vi "Swerve Drive Straight.vi"(0 "Xin":dbl, 3 "Yin":dbl) -> (7 "Xout":dbl, 10 "Yout":dbl)   [LabVIEW 2016]
uses:
  <vilib>/Rock Robotics/WPI/ThirdParty/CanMotor/TalonSRX/WPI_CANTalonSRX_APIControlMode.ctl
  Robot Global Data.vi
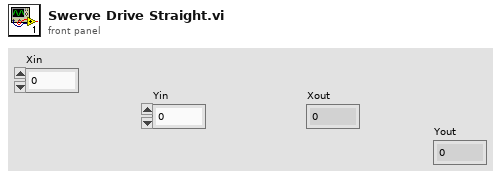
[diagram p1: front panel]
types:
  T1 = enum16{"Start setup globals", "Setup Position control", "run the pid loop", "Change the mode back to PWM", "Finish return values to default"}
  T2 = enum16{"Can ID", "P", "I", "D", "F", "IZone", "RampSpeed", "Fwd speed Limit", "Rev Speed Limit", "InvertDrive"}
  T3 = enum16{"FL Drive Wheel", "FR Drive Wheel", "RL Drive Wheel", "RR Drive Wheel", "FL Steer Wheel", "FR Steer Wheel", "RL Steer Wheel", "RR Steer Wheel"}
  T4 = typedef "WPI_CANTalonSRX_APIControlMode.ctl" = enum8{"Percent VBus", "Speed", "Position", "Slave", "Unchanged / Invalid", "Voltage Compensation", "Current", "Motion Profile", "Motion Magic"}
  T5 = typedef "WPI_MotorControlDeviceRef.ctl" = cluster{"DeviceStatus":errorcluster, "Type":T6, "PWM":cluster{"PWM Channel":T7, "DeadBand":T8}, "CAN":cluster{"Device Number":u8, "SetOutput VI Ref":variant, "GetOutput VI Ref":variant, "Enable VI Ref":variant, "Disable VI Ref":variant, "Data":variant}, "Invert":bool}
  T6 = typedef "WPI_MotorControlType.ctl" = enum16{"PWM", "CAN"}
  T7 = typedef "FPGA_DIOPWMChannel.ctl" = enum8{"PWM 0", "PWM 1", "PWM 2", "PWM 3", "PWM 4", "PWM 5", "PWM 6", "PWM 7", "PWM 8", "PWM 9", "PWM MXP 0", "PWM MXP 1", "PWM MXP 2", "PWM MXP 3", "PWM MXP 4", "PWM MXP 5", "PWM MXP 6", "PWM MXP 7", "PWM MXP 8", "PWM MXP 9", "Invalid"}
  T8 = typedef "WPI_PWMDeadband.ctl" = cluster{"Name":string, "maxPositivePwm":i32, "minPositivePwm":i32, "centerPwm":i32, "maxNegativePwm":i32, "minNegativePwm":i32, "angularRange":u16}
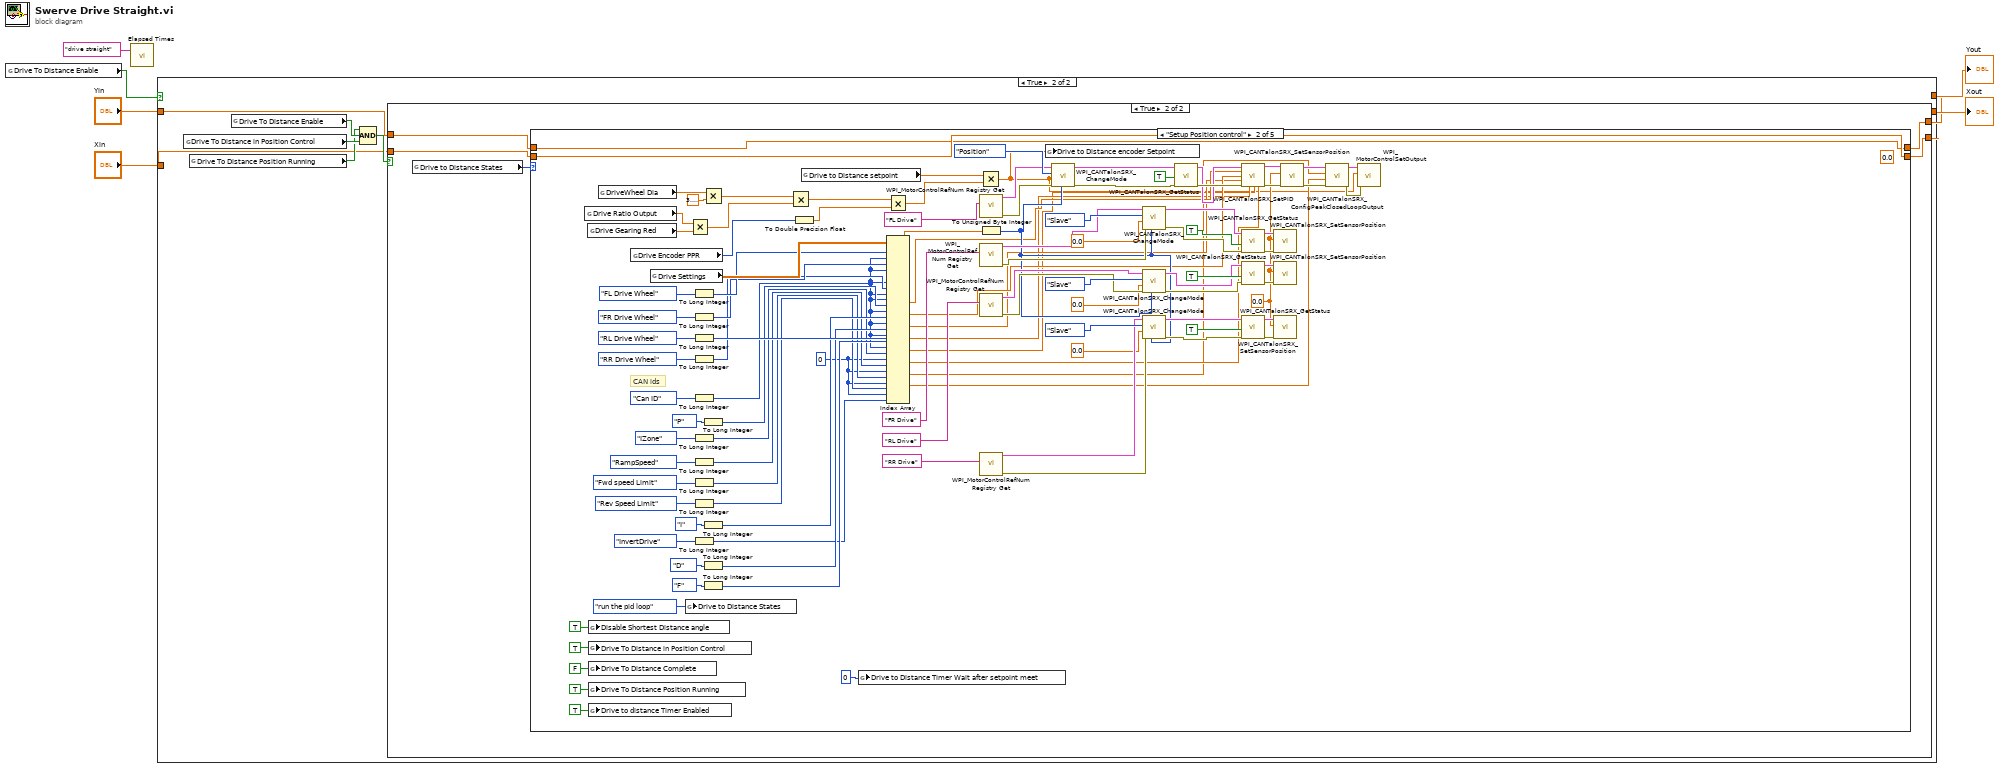
[diagram p0: block diagram]
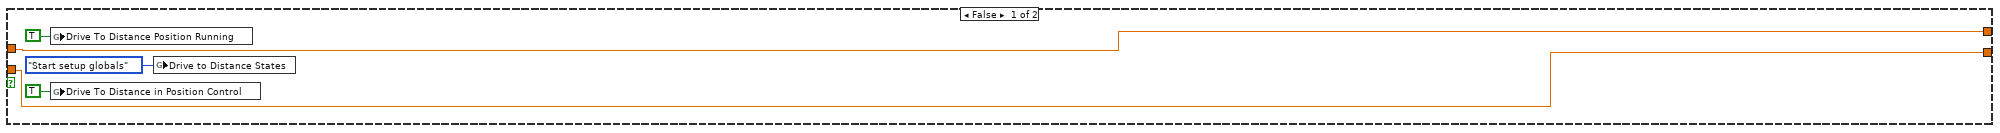
[diagram p3: hidden frame]
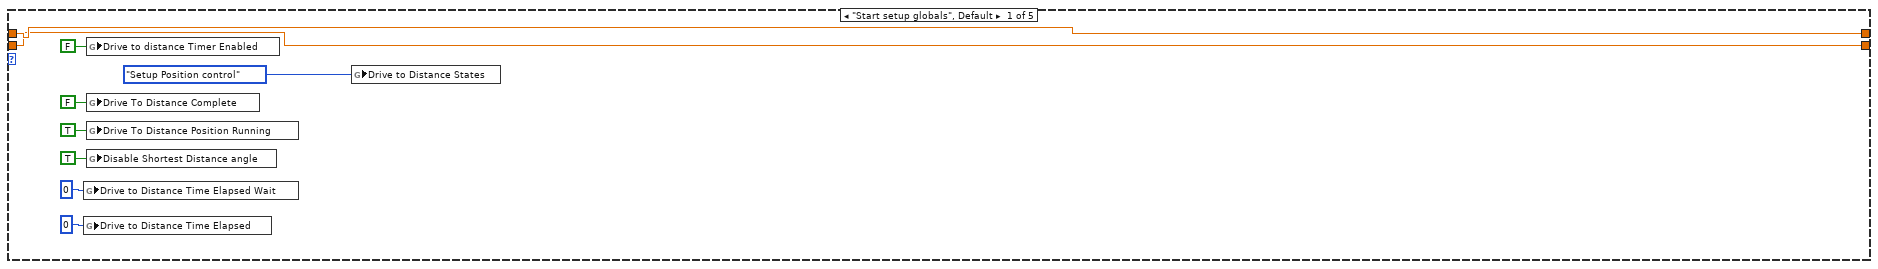
[diagram p4: hidden frame]
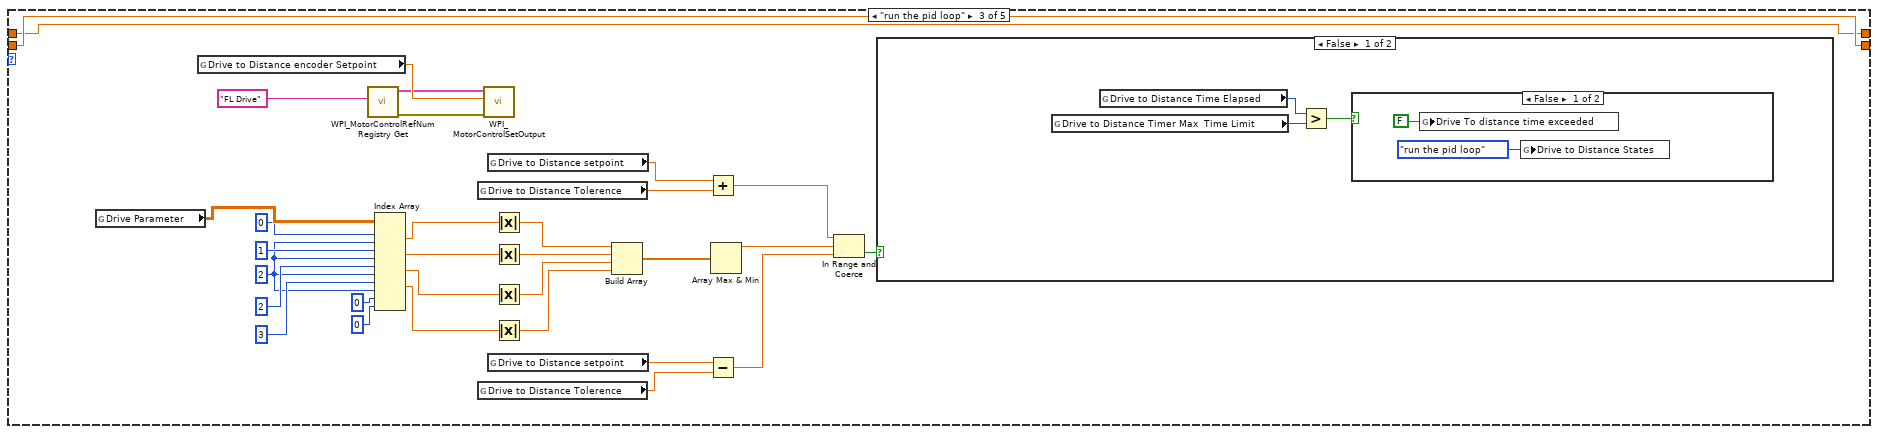
[diagram p5: hidden frame]
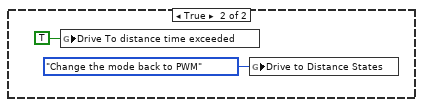
[diagram p6: hidden frame]
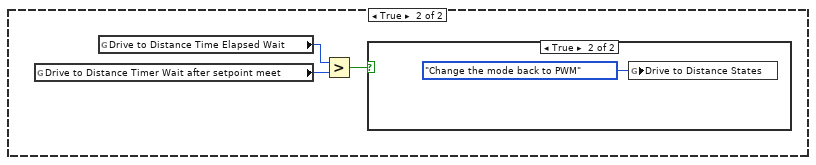
[diagram p7: hidden frame]
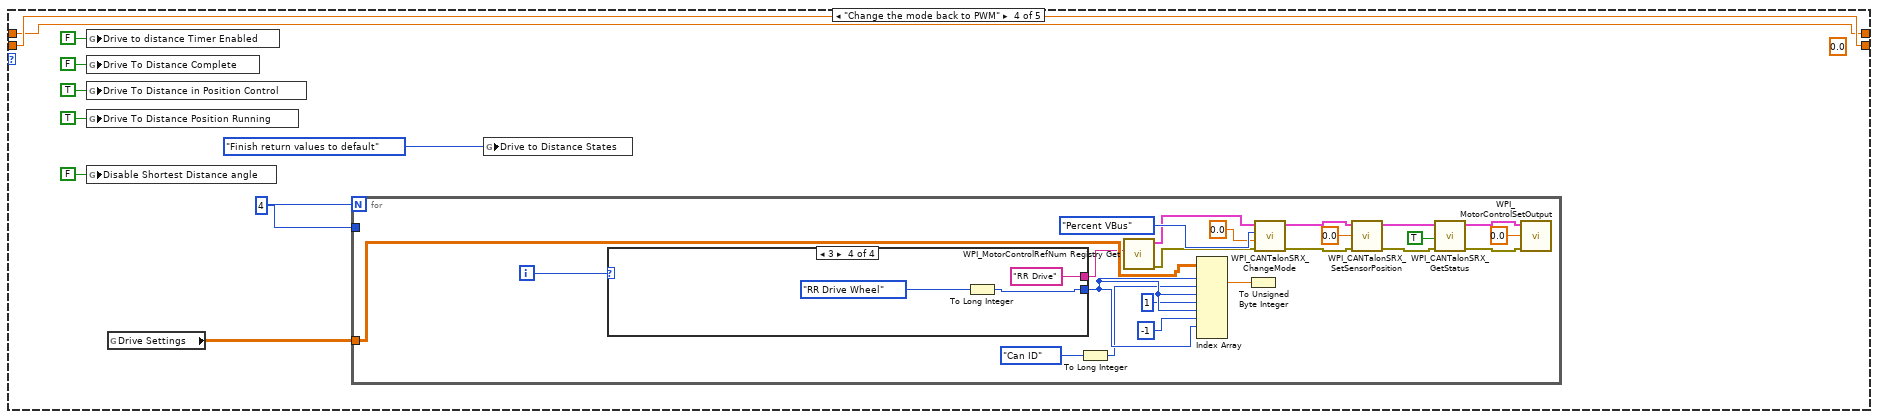
[diagram p9: hidden frame]
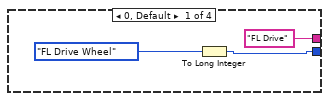
[diagram p10: hidden frame]
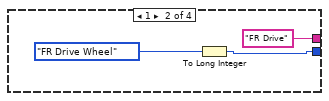
[diagram p11: hidden frame]
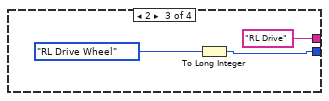
[diagram p12: hidden frame]
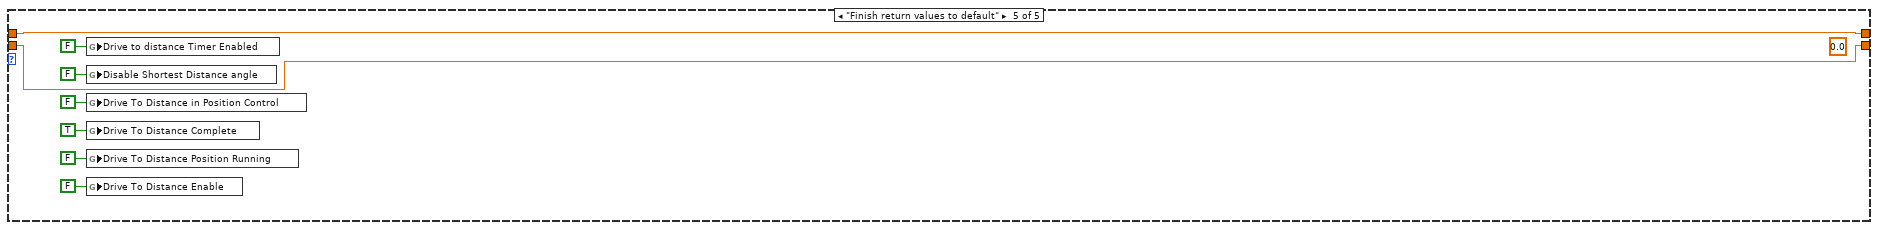
[diagram p13: hidden frame]
diagram:
  n1 = global read "Robot Global Data.vi" "Drive To Distance Enable"() -> (w2:bool)
  n2 = call "Elapsed Times.vi"("Call Name"="drive straight") -> ()  [unwired: 2 in, 1 out]
  n3 = case shown="True" w2 {
    tunnel: [w8 w10] -> w4
    tunnel: "Xin" -> [w8 w12]
    tunnel: [w7 w9] -> w3
    tunnel: "Yin" -> [w7 w11]
    frame False {
    }
    frame True {
      n4 = global read "Robot Global Data.vi" "Drive To Distance in Position Control"() -> (w16:bool)
      n5 = global read "Robot Global Data.vi" "Drive To Distance Position Running"() -> (w14:bool)
      n6 = global read "Robot Global Data.vi" "Drive To Distance Enable"() -> (w15:bool)
      n7 = Compound Arithmetic op=AND(w14, w15, w16) -> (w13:bool)
      n8 = case shown="True" w13 {
        tunnel: w12 -> [w18 w25]
        tunnel: w11 -> [w17 w24]
        tunnel: [w18 w22] -> w10
        tunnel: [w17 w23] -> w9
        frame False {
          n9 = global write "Robot Global Data.vi" "Drive To Distance Position Running"(TRUE ("Drive To Distance Position Running")) -> ()
          n10 = global write "Robot Global Data.vi" "Drive To Distance in Position Control"(TRUE ("Drive To Distance in Position Control")) -> ()
          n11 = global write "Robot Global Data.vi" "Drive to Distance States"(T1."Start setup globals" ("Drive to Distance States")) -> ()
        }
        frame True {
          n12 = global read "Robot Global Data.vi" "Drive to Distance States"() -> (w26:T1)
          n13 = case shown="\"Setup Position control\"" w26 {
            tunnel: w25 -> [w27 w38 w144 w187 w231]
            tunnel: w24 -> [w28 w37 w143 w186 w230]
            tunnel: [w28 w37 w143 w186 w230] -> w23
            tunnel: [w27 w38 w144 w187 w231] -> w22
            frame "Start setup globals", Default {
              n14 = global write "Robot Global Data.vi" "Drive to Distance Time Elapsed Wait"(u32 0 ("Drive to Distance Time Elapsed Wait")) -> ()
              n15 = global write "Robot Global Data.vi" "Drive to Distance Time Elapsed"(u32 0 ("Drive to Distance Time Elapsed")) -> ()
              n16 = global write "Robot Global Data.vi" "Drive to distance Timer Enabled"(FALSE ("Drive To Distance in Position Control")) -> ()
              n17 = global write "Robot Global Data.vi" "Drive To Distance Complete"(FALSE ("Drive To Distance Complete")) -> ()
              n18 = global write "Robot Global Data.vi" "Drive To Distance Position Running"(TRUE ("Drive To Distance Position Running")) -> ()
              n19 = global write "Robot Global Data.vi" "Disable Shortest Distance angle"(TRUE ("Disable Shortest Distance angle")) -> ()
              n20 = global write "Robot Global Data.vi" "Drive to Distance States"(T1."Setup Position control" ("Drive to Distance States")) -> ()
            }
            frame "Setup Position control" {
              (unwired) 0.0 ("Numeric")
              w59 = 0.0 ("New Sensor Position")
              w80 = 0 ("index (row)")
              # "CAN ids"
              n21 = global read "Robot Global Data.vi" "Drive Ratio Output"() -> (w56:dbl)
              n22 = global read "Robot Global Data.vi" "Drive Gearing Red"() -> (w55:dbl)
              n23 = global write "Robot Global Data.vi" "Disable Shortest Distance angle"(TRUE ("Disable Shortest Distance angle")) -> ()
              n24 = global write "Robot Global Data.vi" "Drive To Distance in Position Control"(TRUE ("Drive To Distance in Position Control")) -> ()
              n25 = global write "Robot Global Data.vi" "Drive To Distance Complete"(FALSE ("Drive To Distance Complete")) -> ()
              n26 = global write "Robot Global Data.vi" "Drive To Distance Position Running"(TRUE ("Drive To Distance Position Cont")) -> ()
              n27 = global write "Robot Global Data.vi" "Drive to distance Timer Enabled"(TRUE ("Drive To Distance in Position Control")) -> ()
              n28 = global read "Robot Global Data.vi" "DriveWheel Dia"() -> (w54:dbl)
              n29 = global read "Robot Global Data.vi" "Drive Encoder PPR"() -> (w50:u32)
              n30 = global read "Robot Global Data.vi" "Drive Settings"() -> (w111:dbl[][])
              n31 = global write "Robot Global Data.vi" "Drive to Distance States"(T1."run the pid loop" ("Drive to Distance States")) -> ()
              n32 = Multiply(x=w56, y=w55) -> (x*y=w51:dbl)
              n33 = To Long Integer(number=T3."FL Drive Wheel" ("Swerve Drive Param")) -> (32bit integer=w99:i32)
              n34 = To Long Integer(number=T3."FR Drive Wheel" ("Swerve Drive Param")) -> (32bit integer=w97:i32)
              n35 = To Long Integer(number=T3."RL Drive Wheel" ("Swerve Drive Param")) -> (32bit integer=w98:i32)
              n36 = To Long Integer(number=T3."RR Drive Wheel" ("Swerve Drive Param")) -> (32bit integer=w96:i32)
              n37 = To Long Integer(number=T2."Can ID" ("Enum")) -> (32bit integer=w81:i32)
              n38 = To Long Integer(number=T2."IZone" ("Enum")) -> (32bit integer=w85:i32)
              n39 = To Long Integer(number=T2."RampSpeed" ("Enum")) -> (32bit integer=w86:i32)
              n40 = To Long Integer(number=T2."Fwd speed Limit" ("Enum")) -> (32bit integer=w84:i32)
              n41 = To Long Integer(number=T2."Rev Speed Limit" ("Enum")) -> (32bit integer=w82:i32)
              n42 = To Long Integer(number=T2."InvertDrive" ("Enum")) -> (32bit integer=w83:i32)
              n43 = To Long Integer(number=T2."D" ("Enum")) -> (32bit integer=w93:i32)
              n44 = To Long Integer(number=T2."F" ("Enum")) -> (32bit integer=w92:i32)
              n45 = Multiply(x=w54, y=3.141592653589793) -> (x*y=w52:dbl)
              n46 = To Long Integer(number=T2."P" ("Enum")) -> (32bit integer=w95:i32)
              n47 = To Long Integer(number=T2."I" ("Enum")) -> (32bit integer=w94:i32)
              n48 = Multiply(x=w52, y=w51) -> (x*y=w48:dbl)
              n49 = To Double Precision Float(number=w50) -> (double precision float=w49:dbl)
              n50 = global read "Robot Global Data.vi" "Drive to Distance setpoint"() -> (w46:dbl)
              n51 = global write "Robot Global Data.vi" "Drive to Distance Timer Wait after setpoint meet"(u32 0 ("Drive to Distance Timer Wait after setpoint meet")) -> ()
              n52 = Multiply(x=w48, y=w49) -> (x*y=w47:dbl)
              n53 = Index Array(array=w111, index (row) #1=w99, index (col) #1=w81, index (row) #2=w97, index (col) #2=w81, index (row) #3=w98, index (col) #3=w81, index (row) #4=w96, index (col) #4=w81, index (row) #5=w81, index (col) #5=w95, index (row) #6=w81, index (col) #6=w94, index (row) #7=w81, index (col) #7=w93, index (row) #8=w81, index (col) #8=w92, index (row) #9=w81, index (col) #9=w85, index (row) #10=w80, index (col) #10=w86, index (row) #11=w80, index (col) #11=w84, index (row) #12=w80, index (col) #12=w82, index (row) #13=w80, index (col) #13=w83) -> (element #1=w115:dbl, element #5=w79:dbl, element #6=w78:dbl, element #7=w77:dbl, element #8=w76:dbl, element #9=w75:dbl, element #10=w72:dbl, element #11=w69:dbl, element #12=w68:dbl)  [unwired: 4 out]
              n54 = Multiply(x=w46, y=w47) -> (x*y=w39:dbl)
              n55 = To Unsigned Byte Integer(number=w115) -> (unsigned 8bit integer=w114:u8)
              n56 = call <vilib>:"WPI_MotorControlRefNum Registry Get.vi"("refnum name"="FL Drive") -> ("error out"=w129:errorcluster, "MotorControlDevRef"=w133:T5)  [unwired: 9 in]
              n57 = call <vilib>:"WPI_MotorControlRefNum Registry Get.vi"("refnum name"="FR Drive") -> ("error out"=w128:errorcluster, "MotorControlDevRef"=w132:T5)  [unwired: 9 in]
              n58 = call <vilib>:"WPI_MotorControlRefNum Registry Get.vi"("refnum name"="RL Drive") -> ("error out"=w127:errorcluster, "MotorControlDevRef"=w131:T5)  [unwired: 9 in]
              n59 = call <vilib>:"WPI_MotorControlRefNum Registry Get.vi"("refnum name"="RR Drive") -> ("error out"=w126:errorcluster, "MotorControlDevRef"=w130:T5)  [unwired: 9 in]
              n60 = global write "Robot Global Data.vi" "Drive to Distance encoder Setpoint"(w39) -> ()
              n61 = call <vilib>:"WPI_CANTalonSRX_ChangeMode.vi"("Master Device Number"=w114, "error in (no error)"=w129, "Output"=w39, "Control Mode"=WPI_CANTalonSRX_APIControlMode."Position", "CAN Talon SRX Ref"=w133) -> ("error out"=w125:errorcluster, "CAN Talon SRX Ref"=w124:T5)  [unwired: 5 in]
              n62 = call <vilib>:"WPI_CANTalonSRX_ChangeMode.vi"("Master Device Number"=w114, "error in (no error)"=w128, "Output"=0.0, "Control Mode"=WPI_CANTalonSRX_APIControlMode."Slave", "CAN Talon SRX Ref"=w132) -> ("error out"=w109:errorcluster, "CAN Talon SRX Ref"=w110:T5)  [unwired: 5 in]
              n63 = call <vilib>:"WPI_CANTalonSRX_ChangeMode.vi"("Master Device Number"=w114, "error in (no error)"=w127, "Output"=0.0, "Control Mode"=WPI_CANTalonSRX_APIControlMode."Slave", "CAN Talon SRX Ref"=w131) -> ("error out"=w117:errorcluster, "CAN Talon SRX Ref"=w116:T5)  [unwired: 5 in]
              n64 = call <vilib>:"WPI_CANTalonSRX_ChangeMode.vi"("Master Device Number"=w114, "error in (no error)"=w126, "Output"=0.0, "Control Mode"=WPI_CANTalonSRX_APIControlMode."Slave", "CAN Talon SRX Ref"=w130) -> ("error out"=w118:errorcluster, "CAN Talon SRX Ref"=w119:T5)  [unwired: 5 in]
              n65 = call <vilib>:"WPI_CANTalonSRX_GetStatus.vi"("error in (no error)"=w125, "Clear Sticky Faults"=TRUE, "CAN Talon SRX Ref"=w124) -> ("error out"=w113:errorcluster, "CAN Talon SRX Ref"=w112:T5)  [unwired: 6 in, 1 out]
              n66 = call <vilib>:"WPI_CANTalonSRX_SetPID.vi"("CAN Talon SRX Ref"=w112, "P"=w79, "I"=w78, "D"=w77, "error in (no error)"=w113, "F"=w76, "I Zone"=w75, "Ramp Rate"=w72) -> ("CAN Talon SRX Ref"=w73:T5, "error out"=w74:errorcluster)  [unwired: 6 in]
              n67 = call <vilib>:"WPI_CANTalonSRX_GetStatus.vi"("error in (no error)"=w109, "Clear Sticky Faults"=TRUE, "CAN Talon SRX Ref"=w110) -> ("error out"=w60:errorcluster, "CAN Talon SRX Ref"=w61:T5)  [unwired: 6 in, 1 out]
              n68 = call <vilib>:"WPI_CANTalonSRX_GetStatus.vi"("error in (no error)"=w117, "Clear Sticky Faults"=TRUE, "CAN Talon SRX Ref"=w116) -> ("error out"=w62:errorcluster, "CAN Talon SRX Ref"=w63:T5)  [unwired: 6 in, 1 out]
              n69 = call <vilib>:"WPI_CANTalonSRX_GetStatus.vi"("error in (no error)"=w118, "Clear Sticky Faults"=TRUE, "CAN Talon SRX Ref"=w119) -> ("error out"=w64:errorcluster, "CAN Talon SRX Ref"=w65:T5)  [unwired: 6 in, 1 out]
              n70 = call <vilib>:"WPI_CANTalonSRX_SetSensorPosition.vi"("error in (no error)"=w60, "New Sensor Position"=w59, "CAN Talon SRX Ref"=w61) -> ()  [unwired: 7 in, 2 out]
              n71 = call <vilib>:"WPI_CANTalonSRX_SetSensorPosition.vi"("error in (no error)"=w62, "New Sensor Position"=w59, "CAN Talon SRX Ref"=w63) -> ()  [unwired: 7 in, 2 out]
              n72 = call <vilib>:"WPI_CANTalonSRX_SetSensorPosition.vi"("error in (no error)"=w64, "New Sensor Position"=w59, "CAN Talon SRX Ref"=w65) -> ()  [unwired: 7 in, 2 out]
              n73 = call <vilib>:"WPI_CANTalonSRX_SetSensorPosition.vi"("error in (no error)"=w74, "New Sensor Position"=w59, "CAN Talon SRX Ref"=w73) -> ("error out"=w71:errorcluster, "CAN Talon SRX Ref"=w70:T5)  [unwired: 7 in]
              n74 = call <vilib>:"WPI_CANTalonSRX_ConfigPeakClosedLoopOutput.vi"("error in (no error)"=w71, "Reverse Peak Output"=w68, "Forward Peak Output"=w69, "CAN Talon SRX Ref"=w70) -> ("error out"=w45:errorcluster, "CAN Talon SRX Ref"=w44:T5)  [unwired: 6 in]
              n75 = call <vilib>:"WPI_MotorControlSetOutput.vi"("error in (no error)"=w45, "Output"=w39, "MotorControlDevRef"=w44) -> ()  [unwired: 6 in, 3 out]
            }
            frame "run the pid loop" {
              w170 = 2 ("disabled index (col)")
              n76 = global read "Robot Global Data.vi" "Drive Parameter"() -> (w169:dbl[][])
              n77 = global read "Robot Global Data.vi" "Drive to Distance encoder Setpoint"() -> (w148:dbl)
              n78 = call <vilib>:"WPI_MotorControlRefNum Registry Get.vi"("refnum name"="FL Drive") -> ("error out"=w145:errorcluster, "MotorControlDevRef"=w146:T5)  [unwired: 9 in]
              n79 = Index Array(array=w169, index (row) #1=0 ("disabled index (row)"), index (col) #1=w170, index (row) #2=1 ("index (row)"), index (col) #2=w170, index (row) #3=2 ("index (row)"), index (col) #3=w170, index (row) #4=3 ("index (row)"), index (col) #4=w170, index (row) #5=0 ("index (row)"), index (col) #5=0 ("disabled index (col)")) -> (element #1=w167:dbl, element #2=w164:dbl, element #3=w165:dbl, element #4=w166:dbl)  [unwired: 1 out]
              n80 = global read "Robot Global Data.vi" "Drive to Distance Tolerence"() -> (w156:dbl)
              n81 = global read "Robot Global Data.vi" "Drive to Distance Tolerence"() -> (w154:dbl)
              n82 = call <vilib>:"WPI_MotorControlSetOutput.vi"("error in (no error)"=w145, "Output"=w148, "MotorControlDevRef"=w146) -> ()  [unwired: 6 in, 3 out]
              n83 = global read "Robot Global Data.vi" "Drive to Distance setpoint"() -> (w157:dbl)
              n84 = global read "Robot Global Data.vi" "Drive to Distance setpoint"() -> (w153:dbl)
              n85 = Absolute Value(x=w167) -> (abs(x)=w160:dbl)
              n86 = Absolute Value(x=w164) -> (abs(x)=w161:dbl)
              n87 = Absolute Value(x=w165) -> (abs(x)=w162:dbl)
              n88 = Absolute Value(x=w166) -> (abs(x)=w163:dbl)
              n89 = Build Array(w160, w161, w162, w163) -> (w159:dbl[])
              n90 = Add(x=w157, y=w156) -> (x+y=w155:dbl)
              n91 = Subtract(x=w153, y=w154) -> (x-y=w152:dbl)
              n92 = Array Max & Min(array=w159) -> (max value=w158:dbl)  [unwired: 3 out]
              n93 = In Range and Coerce(upper limit=w155, x=w158, lower limit=w152) -> (In Range?=w151:bool)  [unwired: 1 out]
              n94 = case shown="False" w151 {
                frame False {
                  n95 = global read "Robot Global Data.vi" "Drive to Distance Timer Max  Time Limit"() -> (w175:u32)
                  n96 = global read "Robot Global Data.vi" "Drive to Distance Time Elapsed"() -> (w176:u32)
                  n97 = Greater?(x=w176, y=w175) -> (0:w174:bool)
                  n98 = case shown="False" w174 {
                    frame False {
                      n99 = global write "Robot Global Data.vi" "Drive To distance time exceeded"(FALSE ("Drive To distance time exceeded")) -> ()
                      n100 = global write "Robot Global Data.vi" "Drive to Distance States"(T1."run the pid loop" ("Drive to Distance States")) -> ()
                    }
                    frame True {
                      n101 = global write "Robot Global Data.vi" "Drive To distance time exceeded"(TRUE ("Drive To distance time exceeded")) -> ()
                      n102 = global write "Robot Global Data.vi" "Drive to Distance States"(T1."Change the mode back to PWM" ("Drive to Distance States")) -> ()
                    }
                  }
                }
                frame True {
                  n103 = global read "Robot Global Data.vi" "Drive to Distance Timer Wait after setpoint meet"() -> (w182:u32)
                  n104 = global read "Robot Global Data.vi" "Drive to Distance Time Elapsed Wait"() -> (w183:u32)
                  n105 = Greater?(x=w183, y=w182) -> (0:w181:bool)
                  n106 = case shown="True" w181 {
                    frame False {
                    }
                    frame True {
                      n107 = global write "Robot Global Data.vi" "Drive to Distance States"(T1."Change the mode back to PWM" ("Drive to Distance States")) -> ()
                    }
                  }
                }
              }
            }
            frame "Change the mode back to PWM" {
              (unwired) 0.0 ("Numeric")
              w193 = 4
              n108 = global write "Robot Global Data.vi" "Drive to distance Timer Enabled"(FALSE ("Drive to distance Timer Enabled")) -> ()
              n109 = global write "Robot Global Data.vi" "Drive To Distance Complete"(FALSE ("Drive To Distance Complete")) -> ()
              n110 = global write "Robot Global Data.vi" "Drive To Distance in Position Control"(TRUE ("Drive To Distance in Position Control")) -> ()
              n111 = global write "Robot Global Data.vi" "Drive To Distance Position Running"(TRUE ("Drive To Distance Position Cont")) -> ()
              n112 = global write "Robot Global Data.vi" "Disable Shortest Distance angle"(FALSE ("Disable Shortest Distance angle")) -> ()
              n113 = global read "Robot Global Data.vi" "Drive Settings"() -> (w194:dbl[][])
              n114 = for {
                N: w193 -> [_]
                tunnel: w194 -> [w213]
                tunnel: w193 -> [_]
                i -> [w216]
                n115 = case shown="3" w216 {
                  tunnel: [w219 w221 w224 w227] -> w211
                  tunnel: ["FL Drive" ("refnum name") "FR Drive" ("refnum name") "RL Drive" ("refnum name") "RR Drive" ("refnum name")] -> w201
                  frame 0, Default {
                    n116 = To Long Integer(number=T3."FL Drive Wheel" ("Swerve Drive Param")) -> (32bit integer=w219:i32)
                  }
                  frame 1 {
                    n117 = To Long Integer(number=T3."FR Drive Wheel" ("Swerve Drive Param")) -> (32bit integer=w221:i32)
                  }
                  frame 2 {
                    n118 = To Long Integer(number=T3."RL Drive Wheel" ("Swerve Drive Param")) -> (32bit integer=w224:i32)
                  }
                  frame 3 {
                    n119 = To Long Integer(number=T3."RR Drive Wheel" ("Swerve Drive Param")) -> (32bit integer=w227:i32)
                  }
                }
                n120 = To Long Integer(number=T2."Can ID" ("Enum")) -> (32bit integer=w210:i32)
                n121 = call <vilib>:"WPI_MotorControlRefNum Registry Get.vi"("refnum name"=w201) -> ("error out"=w203:errorcluster, "MotorControlDevRef"=w202:T5)  [unwired: 9 in]
                n122 = Index Array(array=w213, index (row) #1=w211, index (col) #1=w210, index (row) #2=w211, index (col) #2=1 ("index (col)"), index (row) #3=w211, index (col) #3=-1 ("index (col)"), index (row) #4=w211) -> (element #1=w214:dbl)  [unwired: 1 in, 3 out]
                n123 = To Unsigned Byte Integer(number=w214) -> ()  [unwired: 1 out]
                n124 = call <vilib>:"WPI_CANTalonSRX_ChangeMode.vi"("error in (no error)"=w203, "Output"=0.0, "Control Mode"=WPI_CANTalonSRX_APIControlMode."Percent VBus", "CAN Talon SRX Ref"=w202) -> ("error out"=w200:errorcluster, "CAN Talon SRX Ref"=w199:T5)  [unwired: 6 in]
                n125 = call <vilib>:"WPI_CANTalonSRX_SetSensorPosition.vi"("error in (no error)"=w200, "New Sensor Position"=0.0, "CAN Talon SRX Ref"=w199) -> ("error out"=w208:errorcluster, "CAN Talon SRX Ref"=w209:T5)  [unwired: 7 in]
                n126 = call <vilib>:"WPI_CANTalonSRX_GetStatus.vi"("error in (no error)"=w208, "Clear Sticky Faults"=TRUE, "CAN Talon SRX Ref"=w209) -> ("error out"=w197:errorcluster, "CAN Talon SRX Ref"=w198:T5)  [unwired: 6 in, 1 out]
                n127 = call <vilib>:"WPI_MotorControlSetOutput.vi"("error in (no error)"=w197, "Output"=0.0, "MotorControlDevRef"=w198) -> ()  [unwired: 6 in, 3 out]
              }
              n128 = global write "Robot Global Data.vi" "Drive to Distance States"(T1."Finish return values to default" ("Drive to Distance States")) -> ()
            }
            frame "Finish return values to default" {
              (unwired) 0.0 ("Numeric")
              n129 = global write "Robot Global Data.vi" "Drive to distance Timer Enabled"(FALSE ("Drive to distance Timer Enabled")) -> ()
              n130 = global write "Robot Global Data.vi" "Disable Shortest Distance angle"(FALSE ("Disable Shortest Distance angle")) -> ()
              n131 = global write "Robot Global Data.vi" "Drive To Distance in Position Control"(FALSE ("Drive To Distance in Position Control")) -> ()
              n132 = global write "Robot Global Data.vi" "Drive To Distance Complete"(TRUE ("Drive To Distance Complete")) -> ()
              n133 = global write "Robot Global Data.vi" "Drive To Distance Position Running"(FALSE ("Drive To Distance Position Cont")) -> ()
              n134 = global write "Robot Global Data.vi" "Drive To Distance Enable"(FALSE ("Drive To Distance Enable")) -> ()
            }
          }
        }
      }
    }
  }
  "Yout" <- w3
  "Xout" <- w4
